vi "Unpack Spectra.vi"(0 "packed spectra":dbl[][](array[numeric]), 4 "spectra info":string[][](array[string])) -> (14 "spectra":cluster{"f0":dbl, "df":dbl, "magnitude":dbl[]}[](array[cluster]) {"magnitude" format="%.2p"; "df" format="%.2p"; "f0" format="%.2p"}, 18 "spectrum info":T1[](array[typedef]) {"x-axis units" items=["Time (s)"=0, "Frequency-CB (Hz)"=1, "Frequency-CPB (Hz)"=1248, "Frequency-Arbitrary (Hz)"=2357, "Quefrency (s)"=2, "Revolutions (rev)"=3, "Order"=4, "Speed (RPM)"=11, "Speed (rad/s)"=21, "Index"=65535]; "weighting filter" items=["Linear", "A-weighting", "B-weighting", "C-weighting", "ITU-R 468-4", "Dolby", "CCITT", "C-message", "Wb", "Wc", "Wd", "We", "Wf", "Wh", "Wj", "Wk", "Wm", "AES17 20 kHz lowpass", "AES17 40 kHz lowpass", "AES17 20 kHz highpass", "AES17 40 kHz highpass"]; "dB reference [EU]" format="%.2f"; "engineering units" items=["custom..."=0, "V"=1, "A"=21, "C"=30, "pC"=31, "s"=32, "-"=29, "Pa"=2, "N"=20, "g"=3, "m/s^2"=4, "m/s"=5, "m"=6, "mm/s"=12, "mm"=13, "micron/s"=14, "micron"=15, "in/s^2"=7, "in/s"=8, "in"=9, "mil/s"=10, "mil"=11, "rad/s^2"=16, "rad/s"=17, "rad"=18, "deg/s^2"=26, "deg/s"=27, "deg"=28, "RPM"=22, "cycle/s^2"=23, "Hz"=24, "cycle"=25, "strain"=19]; "spectral info"."window" items=["None "=0, "Hanning"=1, "Hamming"=2, "Blackman-Harris"=3, "Exact Blackman"=4, "Blackman"=5, "Flat Top"=6, "4 Term B-Harris "=7, "7 Term B-Harris"=8, "Low Sidelobe"=9, "Force - Exponential"=10, "Gaussian"=62]})   [LabVIEW 2024, in "Dynamic Signal Acquisition (Interactive) UI.lvlib"]
uses:
  <vilib>/addons/_NISVFA/_Shared subVIs/Controls/svc_Spectrum Info.ctl
  <vilib>/addons/_NISVFA/_Shared subVIs/Controls/svc_X-Axis Units.ctl
  <vilib>/addons/_NISVFA/_Shared subVIs/Controls/svc_Spectrum Type.ctl
  <vilib>/addons/_NISVFA/_Shared subVIs/Controls/svc_Engineering Units Text Ring.ctl
  <vilib>/addons/_NISVFA/_Shared subVIs/Controls/svc_Weighting Filter Text Ring.ctl
  <vilib>/addons/_NISVFA/_Shared subVIs/Controls/svc_Complimentary Spectrum Units.ctl
  Dynamic Signal Acquisition (Interactive) UI.lvlib
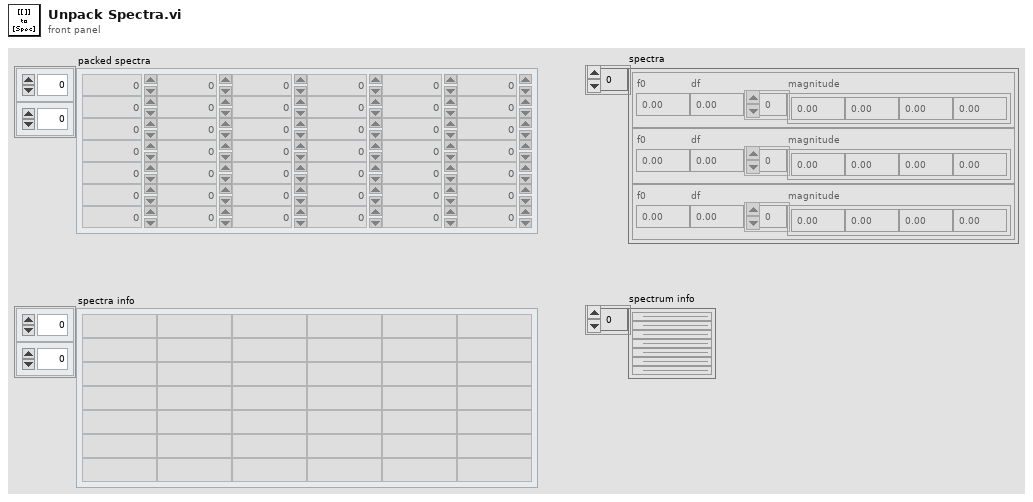
[diagram p1: front panel]
types:
  T1 = typedef "svc_Spectrum Info.ctl" = cluster{"channel name":string, "description":string, "x-axis units":T2, "spectral info":cluster{"spectrum type":T3, "linear/dB":enum16{"linear", "dB"}, "window":u16, "window size":i32, "FFT size":i32}, "engineering units":T4, "custom label":string, "dB reference [EU]":dbl, "peak units":enum16{"rms", "peak", "peak-peak"}, "weighting filter":T5, "spectral density?":bool, "unit label":string, "spectrum skewed?":bool, "complimentary spectrum units":T6}
  T2 = typedef "svc_X-Axis Units.ctl" = u16
  T3 = typedef "svc_Spectrum Type.ctl" = enum16{"FFT Spectrum [complex]", "Amplitude [Magnitude]", "Power [Magnitude^2]", "Cross Spectrum [complex]", "Frequency Response [Complex]"}
  T4 = typedef "svc_Engineering Units Text Ring.ctl" = u16
  T5 = typedef "svc_Weighting Filter Text Ring.ctl" = u16
  T6 = typedef "svc_Complimentary Spectrum Units.ctl" = enum16{"none", "radians", "degrees", "cycles", "imaginary"}
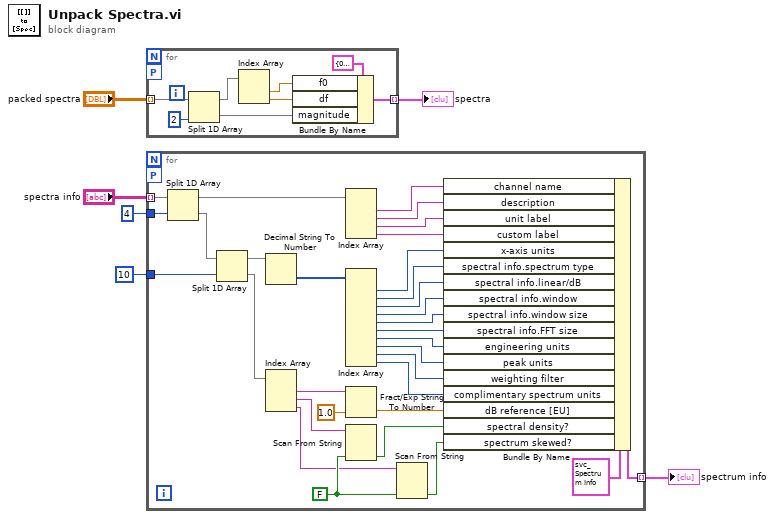
[diagram p0: block diagram]
diagram:
  n1 = for {
    workers-P: _ -> [_]
    tunnel: "packed spectra" -> [w13] mode=indexing
    tunnel: [w7] -> w5 mode=indexing
    n2 = Split 1D Array(array=w13, index=2) -> (first subarray=w12:dbl[], second subarray=w10:dbl[])
    n3 = Index Array(array=w12) -> (element #1=w8:dbl, element #2=w9:dbl)  [unwired: 2 in]
    n4 = Bundle By Name(cluster=cluster{"f0":dbl, "df":dbl, "magnitude":dbl[]} {"f0"=0.0, "df"=0.0, "magnitude"=[]}, "f0"=w8, "df"=w9, "magnitude"=w10) -> (w7:cluster{"f0":dbl, "df":dbl, "magnitude":dbl[]})
  }
  "spectra" <- w5
  n5 = for {
    tunnel: "spectra info" -> [w45] mode=indexing
    tunnel: 4 ("index") -> [w39]
    tunnel: 10 ("index") -> [w38]
    tunnel: [w17] -> w1 mode=indexing
    workers-P: _ -> [_]
    w20 = FALSE
    n6 = Split 1D Array(array=w45, index=w39) -> (first subarray=w40:string[], second subarray=w15:string[])
    n7 = Split 1D Array(array=w15, index=w38) -> (first subarray=w37:string[], second subarray=w35:string[])
    n8 = Decimal String To Number(string=w37) -> (number=w36:i32[])  [unwired: 2 in, 1 out]
    n9 = Index Array(array=w35) -> (element #1=w24:string, element #2=w21:string, element #3=w16:string)  [unwired: 3 in]
    n10 = Index Array(array=w40) -> (element #1=w44:string, element #2=w43:string, element #3=w42:string, element #4=w41:string)  [unwired: 4 in]
    n11 = Index Array(array=w36) -> (element #1=w34:i32, element #2=w33:i32, element #3=w32:i32, element #4=w31:i32, element #5=w30:i32, element #6=w29:i32, element #7=w28:i32, element #8=w27:i32, element #9=w26:i32, element #10=w25:i32)  [unwired: 10 in]
    n12 = Fract/Exp String To Number(string=w24, default (0 dbl)=1.0 ("default (0 DBL)")) -> (number=w22:dbl)  [unwired: 2 in, 1 out]
    n13 = Scan From String(input string=w21, default 1=w20) -> (output 1=w18:bool)  [unwired: 3 in, 3 out]
    n14 = Scan From String(input string=w16, default 1=w20) -> (output 1=w19:bool)  [unwired: 3 in, 3 out]
    n15 = Bundle By Name(cluster=T1 {"channel name"="", "description"="", "x-axis units"=0, "spectral info"={"spectrum type"=enum."Power [Magnitude^2]", "linear/dB"=enum."linear", "window"=0, "window size"=0, "FFT size"=0}, "engineering units"=0, "custom label"="", "dB reference [EU]"=0.0, "peak units"=enum."rms", "weighting filter"=0, "spectral density?"=FALSE, "unit label"="", "spectrum skewed?"=FALSE, "complimentary spectrum units"=enum."none"} ("spectrum info"), "channel name"=w44, "description"=w43, "unit label"=w42, "custom label"=w41, "x-axis units"=w34, "spectral info.spectrum type"=w33, "spectral info.linear/dB"=w32, "spectral info.window"=w31, "spectral info.window size"=w30, "spectral info.FFT size"=w29, "engineering units"=w28, "peak units"=w27, "weighting filter"=w26, "complimentary spectrum units"=w25, "dB reference [EU]"=w22, "spectral density?"=w18, "spectrum skewed?"=w19) -> (w17:T1)
  }
  "spectrum info" <- w1
